vi "Set Icon Source Path INI.vi"(8 "error in":errorcluster, 10 "Icon source dir":path, 11 "config.ini path":path) -> (0 "error out":errorcluster, 3 "config.ini path dup":path)   [LabVIEW 2012]
uses:
  INI_source.ctl
  <vilib>/Utility/config.llb/NI_LVConfig.lvlib
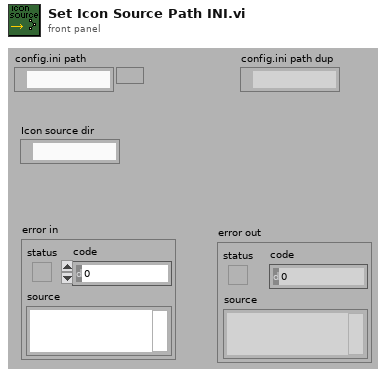
[diagram p1: front panel]
types:
  T1 = typedef "INI_source.ctl" = cluster{"Icon source":path}
  T2 = typedef "NI_LVConfig.lvlib/Config Data RefNum.ctl" = refnum<k1>
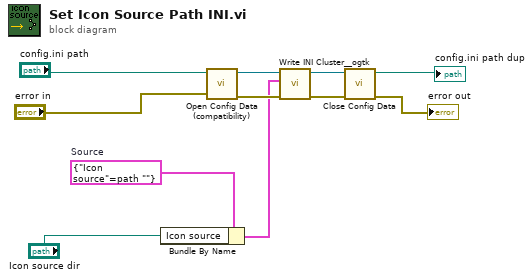
[diagram p0: block diagram]
diagram:
  w7 = T1 {"Icon source"=path ""}  # Source
  n1 = Bundle By Name(cluster=w7, "Icon source"="Icon source dir") -> (w6:T1)
  n2 = call <vilib>:"Open Config Data (compatibility).vi"("error in (no error)"="error in", "configuration file path"="config.ini path") -> ("error out"=w11:errorcluster, "refnum"=w10:T2)  [unwired: 7 in, 1 out]
  n3 = call <userlib>:"Write INI Cluster__ogtk.vi"("error in (no error)"=w11, "INI Fomatted Cluster"=w6, "refnum"=w10) -> ("error out"=w4:errorcluster, "dup refnum"=w5:T2)  [unwired: 1 in, 6 out]
  n4 = call <vilib>:"Close Config Data.vi"("error in (no error)"=w4, "refnum"=w5) -> ("error out"=→"error out":errorcluster, "file path"=→"config.ini path dup":path)  [unwired: 1 in, 7 out]
